vi "Test - Set Player Positions.vi"   [LabVIEW 2018, in "Camera.lvclass"]
uses:
  Camera.lvclass
  LabSDL2/Source/Libraries/SDL2 Utility/Point (I32).ctl
  Camera.lvclass/Camera.ctl
  <vilib>/addons/_JKI Toolkits/Caraya/classes/Test/Test.lvclass
  LabSDL2/Source/Libraries/SDL2 Utility/SDL2 Utility.lvlib
  <vilib>/addons/_JKI Toolkits/Caraya/classes/Assert/Assert.lvclass
types:
  T1 = typedef "SDL2 Utility.lvlib/Point (I32).ctl" = cluster{"x":i32, "y":i32}
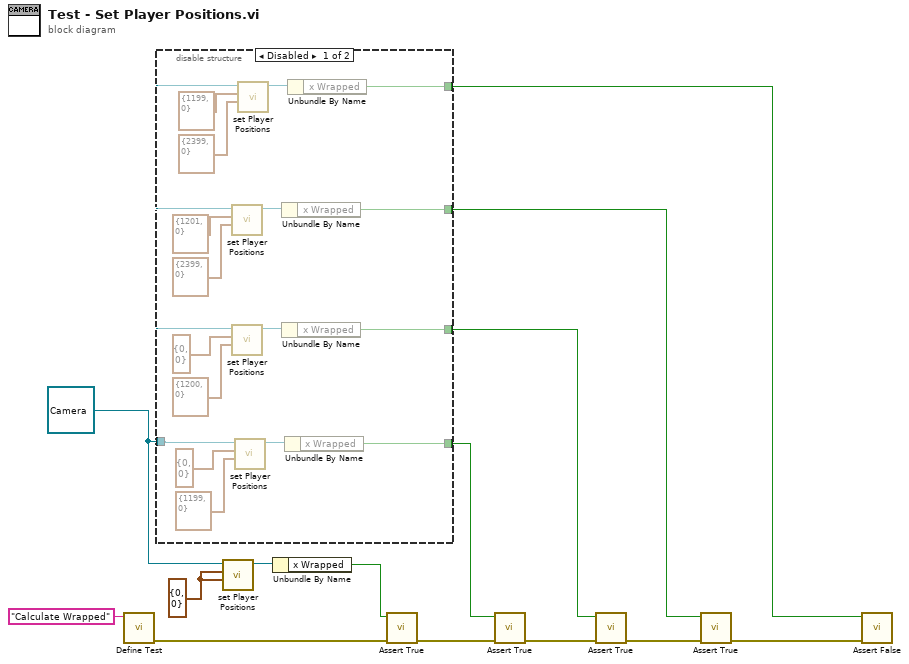
[diagram p0: block diagram]
diagram:
  w2 = refnum<class "Camera.lvclass"> refnum ("Camera.lvclass")
  w13 = T1 {"x"=0, "y"=0} ("Player 1 World Position")
  n1 = call <vilib>:"Define Test.vi"("Label (VI Title)"="Calculate Wrapped") -> ("error out"=w11:errorcluster)  [unwired: 10 in]
  n2 = disable-structure shown="Disabled" {
    disable-tunnel: [w28 _] -> w8
    disable-tunnel: [w24 _] -> w6
    disable-tunnel: [w20 _] -> w5
    disable-tunnel: w2 -> [w16 _]
    disable-tunnel: [w15 _] -> w1
    frame Disabled {
      n3 = call "set Player Positions.vi"("Player 2 Position"=T1 {"x"=2399, "y"=0} ("Player 1 World Position"), "Player 1 Position"=T1 {"x"=1201, "y"=0} ("Player 1 World Position"), "Camera in"=w16) -> ("Camera out"=w23:refnum<class "Camera.lvclass">)  [unwired: 8 in]
      n4 = call "set Player Positions.vi"("Player 2 Position"=T1 {"x"=1200, "y"=0} ("Player 1 World Position"), "Player 1 Position"=T1 {"x"=0, "y"=0} ("Player 1 World Position"), "Camera in"=w16) -> ("Camera out"=w25:refnum<class "Camera.lvclass">)  [unwired: 8 in]
      n5 = call "set Player Positions.vi"("Player 2 Position"=T1 {"x"=1199, "y"=0} ("Player 1 World Position"), "Player 1 Position"=T1 {"x"=0, "y"=0} ("Player 1 World Position"), "Camera in"=w16) -> ("Camera out"=w31:refnum<class "Camera.lvclass">)  [unwired: 8 in]
      n6 = call "set Player Positions.vi"("Player 2 Position"=T1 {"x"=2399, "y"=0} ("Player 1 World Position"), "Player 1 Position"=T1 {"x"=1199, "y"=0} ("Player 1 World Position"), "Camera in"=w16) -> ("Camera out"=w17:refnum<class "Camera.lvclass">)  [unwired: 8 in]
      n7 = Unbundle By Name(w23) -> ("x Wrapped"=w20:bool)
      n8 = Unbundle By Name(w25) -> ("x Wrapped"=w24:bool)
      n9 = Unbundle By Name(w31) -> ("x Wrapped"=w28:bool)
      n10 = Unbundle By Name(w17) -> ("x Wrapped"=w15:bool)
    }
    frame Enabled {
    }
  }
  n11 = call "set Player Positions.vi"("Player 2 Position"=w13, "Player 1 Position"=w13, "Camera in"=w2) -> ("Camera out"=w12:refnum<class "Camera.lvclass">)  [unwired: 8 in]
  n12 = Unbundle By Name(w12) -> ("x Wrapped"=w10:bool)
  n13 = call <vilib>:"Assert True.vi"("error in (no error)"=w11, "True?"=w10) -> ("error out"=w9:errorcluster)  [unwired: 9 in]
  n14 = call <vilib>:"Assert True.vi"("error in (no error)"=w9, "True?"=w8) -> ("error out"=w7:errorcluster)  [unwired: 9 in]
  n15 = call <vilib>:"Assert True.vi"("error in (no error)"=w7, "True?"=w6) -> ("error out"=w4:errorcluster)  [unwired: 9 in]
  n16 = call <vilib>:"Assert True.vi"("error in (no error)"=w4, "True?"=w5) -> ("error out"=w3:errorcluster)  [unwired: 9 in]
  n17 = call <vilib>:"Assert False.vi"("error in (no error)"=w3, "False?"=w1) -> ()  [unwired: 9 in, 1 out]
